vi "Kinesis - BPC301 - Waveform LUT.vi"() -> ()   [LabVIEW 2012]
uses:
  U:/Kinesis LabVIEW Website Examples/Thorlabs.MotionControl.Controls.dll
  Thorlabs.MotionControl.Controls.dll
  U:/Kinesis LabVIEW Website Examples/Thorlabs.MotionControl.GenericPiezoCLI.dll
  Thorlabs.MotionControl.GenericPiezoCLI.dll
  <vilib>/measure/NI_MABase.lvlib
  U:/Kinesis LabVIEW Website Examples/Thorlabs.MotionControl.Benchtop.PiezoCLI.dll
  Thorlabs.MotionControl.Benchtop.PiezoCLI.dll
panel:
  in  "?":bool
  in  "?":bool
  in  "Milliseconds to Stop":u32=10000
  out "Sine Wave Array":dbl[](array[numeric])
  in  "Peak Voltage":dbl=5.0
  in  "SerialNumber":string
  in  "NumberOfCycles":u32
  in  "Mode":i16(ring)=1 items=["Continuous"=1, "Fixed"=2, "OutputTrigEnable"=4, "InputTrigEnable"=8, "OutputTrigSenseHigh"=16, "InputTrigSenseHigh"=32, "OutputGated"=64, "OutputTrigRepeat"=128]
  in  "LUTValDelay":u32=10
  in  "PostCycleDelay":u32=5
  in  "PreCycleDelay":u32=5
  in  "BenchtopPiezoControl":refnum<k24>(container)
  # "Notes:"
  # "- Ensure that the appropriate .DLLs are copied into your Project Folder. Check that the correct bit type are used depending on your version of LabVIEW\ni.e. 32-bit or 64-bit.\n\n\n\n\n\n\n\n\n\n\n\n\n\n\n- Open the example VI through the LabVIEW Project Explorer to correctly load the User Interface from Thorlabs.MotionControl.Controls.dll."
  # "Thorlabs Hardware: BPC301 - 1-Channel Benchtop Piezo Controller\nhttps://www.thorlabs.com/newgrouppage9.cfm?objectgroup_id=1912&pn=BPC301\n\nDescription: This VI will enable you to make use of the LUTWave Functionality available to Piezo actuated device. \nTaking advantage of the built-in Sine Waveform.vi of LabVIEW, we produce an array of sine wave component values, \nscaled by the Peak Voltage parameter below to produce our waveform. The sine wave period is represented by 50 indexed values in the array.\nUsers are then prompted to select parameters of the LUTWaveParams() struct below the UI before initiating the waveform by clicking 'GO'.\nThe below settings will output the waveform continuously until a 10 second timer has elapsed.\n\nInstructions: \n1) Connect your KPZ101 device to your PC & ensure it is powered on & the Output Enabled. \nFor full device setup, the device product manual can be found on our website here. - https://www.thorlabs.com/thorproduct.cfm?partnumber=BPC301\n2) Enter the device serial number below.\n3) Click 'Run' in the LabVIEW Toolbar.\n4) Assign a timer for 'Milliseconds to Stop' as a timeout for when the Waveform should stop.\n5) Assign Parameters to the Waveform & then Click 'GO' - this will print the sine wave array to the front panel & then start the waveform output.\n6) Click 'STOP' to end the program."
  # "Example Image of .NET Controller - VI opened via Project Explorer/ not opened via Project Explorer"
  # "VI Not Opened via Project Explorer"
  # "VI Opened via Project Explorer"
  # "Time before next cycle starts"
  # "- To explore the range of methods available, please visit the .NET API, included with your Kinesis software.\n\n- For tips on building your own VIs with Thorlabs Motion Control Hardware, please see our LabVIEW Guide here.\nhttps://www.thorlabs.com/newgrouppage9.cfm?objectgroup_id=10285"
  # "Number of times to repeat cycles"
  # "Time between output updates"
  # "Time after cycle finishes"
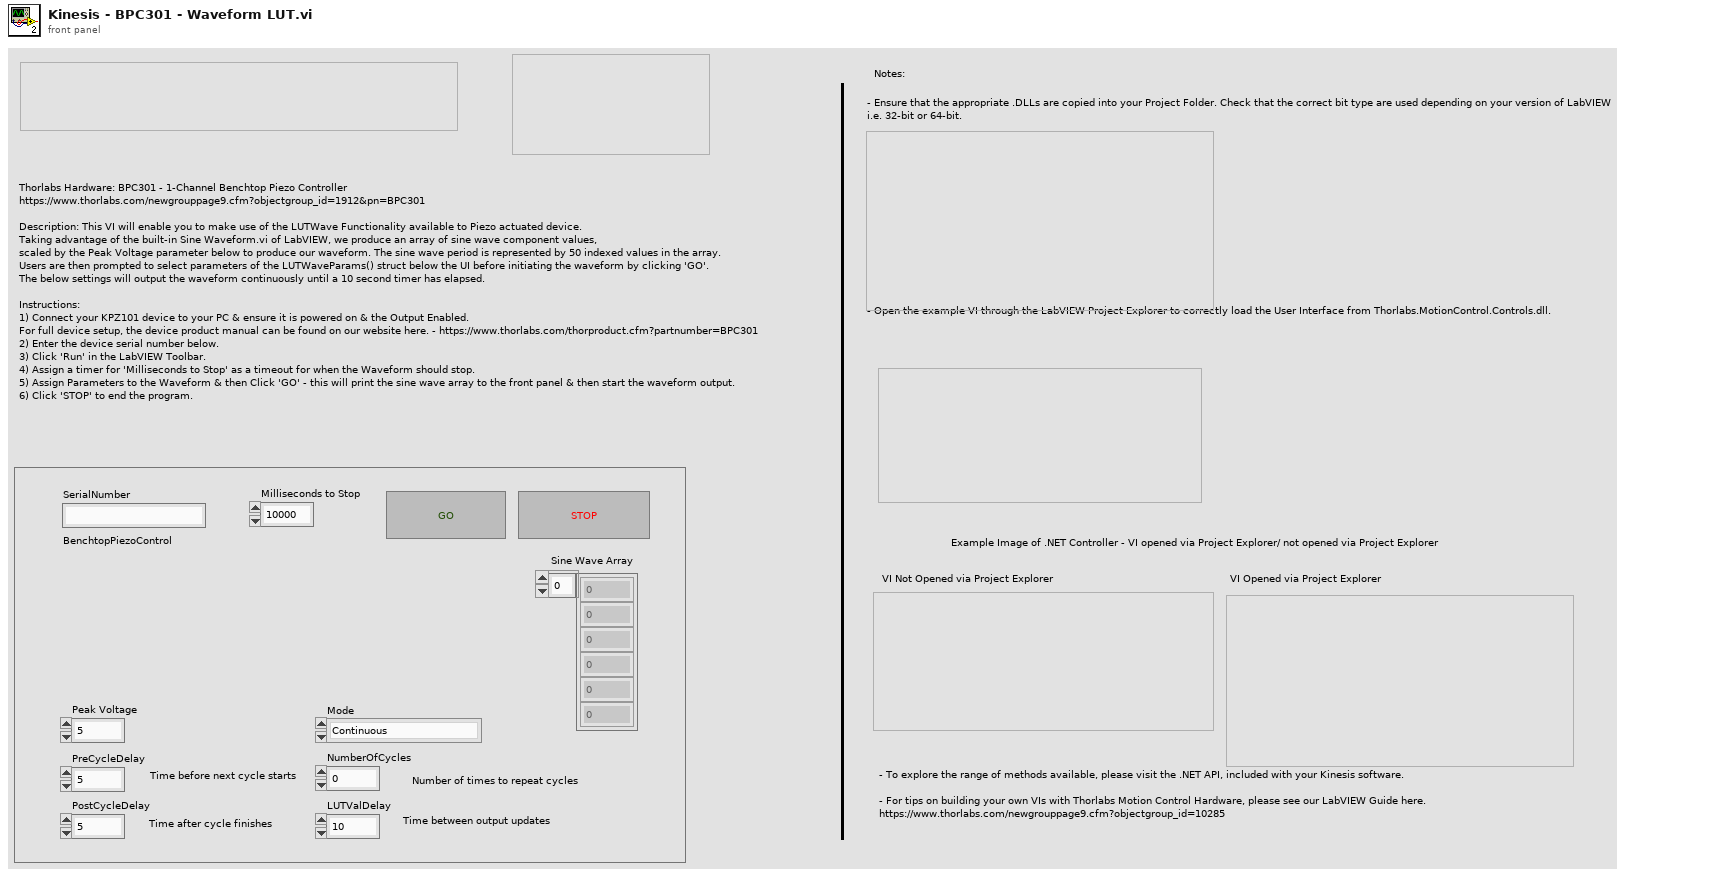
[diagram p1: front panel]
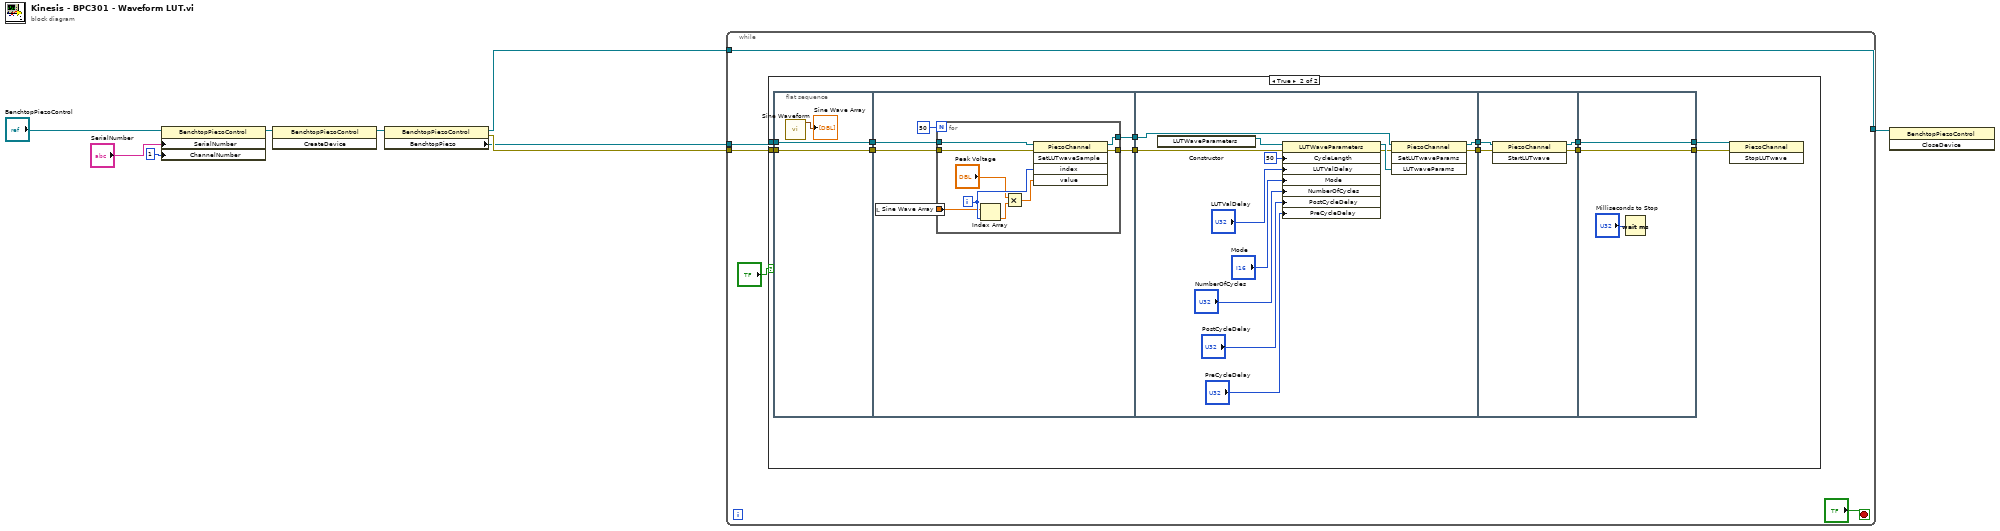
[diagram p0: block diagram]
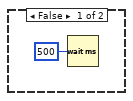
[diagram p2: hidden frame]
diagram:
  n1 = property class="BenchtopPiezoControl"(reference="BenchtopPiezoControl", "SerialNumber"="SerialNumber", "ChannelNumber"=1) -> (reference out=w6:refnum<k24>)  [unwired: 1 in, 1 out]
  n2 = invoke class="BenchtopPiezoControl" method="CreateDevice"(reference=w6) -> (reference out=w5:refnum<k24>)  [unwired: 2 in, 2 out]
  n3 = property class="BenchtopPiezoControl"(reference=w5) -> (reference out=w2:refnum<k24>, error out=w4:errorcluster, "BenchtopPiezo"=w3:refnum<k24>)  [unwired: 1 in]
  n4 = while {
    tunnel: w4 -> [w14]
    tunnel: w3 -> [w13]
    tunnel: [w12] -> w1
    tunnel: w2 -> [w12]
    stop <- "?" stop-if-true
    n5 = case shown="True" "?" {
      tunnel: w13 -> [_ w19]
      tunnel: w14 -> [_ w18]
      frame False {
        n6 = Wait (ms)(milliseconds to wait=u32 500) -> ()  [unwired: 1 out]
      }
      frame True {
        n7 = flat-sequence {
          tunnel: w18 -> [w29]
          tunnel: w19 -> [w30]
          tunnel: [w30] -> w27
          tunnel: [w29] -> w26
          tunnel: [w34] -> w25
          tunnel: [w32] -> w24
          tunnel: w27 -> [w35]
          tunnel: w26 -> [w33]
          tunnel: [w50] -> w23
          tunnel: w25 -> [w51]
          tunnel: w24 -> [w49]
          tunnel: [w47] -> w22
          tunnel: w23 -> [w62]
          tunnel: w22 -> [w60]
          tunnel: [w61] -> w21
          tunnel: [w59] -> w20
          tunnel: [w64] -> w16
          tunnel: [w65] -> w17
          tunnel: w21 -> [w65]
          tunnel: w20 -> [w64]
          frame #0 {
            n8 = call <vilib>:"Sine Waveform.vi"() -> ("signal out"=→"Sine Wave Array":waveform(dbl))  [unwired: 10 in, 1 out]
          }
          frame #1 {
            n9 = local read "Sine Wave Array"() -> (w31:dbl[])
            n10 = for {
              N: 50 -> [_]
              tunnel: w35 -> [w42]
              tunnel: [w41] -> w34
              tunnel: w33 -> [w39]
              tunnel: [w38] -> w32
              tunnel: w31 -> [w37]
              i -> [w45]
              n11 = Index Array(array=w37, index=w45) -> (element=w44:dbl)
              n12 = Multiply(x="Peak Voltage", y=w44) -> (x*y=w40:dbl)
              n13 = invoke class="PiezoChannel" method="SetLUTwaveSample"(reference=w42, error in=w39, "index"=w45, "value"=w40) -> (reference out=w41:refnum<k24>, error out=w38:errorcluster)  [unwired: 1 in, 3 out]
            }
          }
          frame #2 {
            n14 = constructor class="LUTWaveParameters"() -> (reference out=w53:refnum<k24>)  [unwired: 3 in, 2 out]
            n15 = property class="LUTWaveParameters"(reference=w53, error in=w49, "CycleLength"=i16 50, "LUTValDelay"="LUTValDelay", "Mode"="Mode", "NumberOfCycles"="NumberOfCycles", "PostCycleDelay"="PostCycleDelay", "PreCycleDelay"="PreCycleDelay") -> (reference out=w52:refnum<k24>, error out=w48:errorcluster)
            n16 = invoke class="PiezoChannel" method="SetLUTwaveParams"(reference=w51, error in=w48, "LUTwaveParams"=w52) -> (reference out=w50:refnum<k24>, error out=w47:errorcluster)  [unwired: 1 in, 2 out]
          }
          frame #3 {
            n17 = invoke class="PiezoChannel" method="StartLUTwave"(reference=w62, error in=w60) -> (reference out=w61:refnum<k24>, error out=w59:errorcluster)  [unwired: 1 in, 1 out]
          }
          frame #4 {
            n18 = Wait (ms)(milliseconds to wait="Milliseconds to Stop") -> ()  [unwired: 1 out]
          }
        }
        n19 = invoke class="PiezoChannel" method="StopLUTwave"(reference=w17, error in=w16) -> ()  [unwired: 1 in, 3 out]
      }
    }
  }
  n20 = invoke class="BenchtopPiezoControl" method="CloseDevice"(reference=w1) -> ()  [unwired: 2 in, 3 out]
